vi "data-logging-test.vi"() -> ()   [LabVIEW 2023]
panel:
  out "error IO":errorcluster
  out "Datapoint 1":i32
  in  "Log File Name":path=path "log-00"
  in  "Start":bool
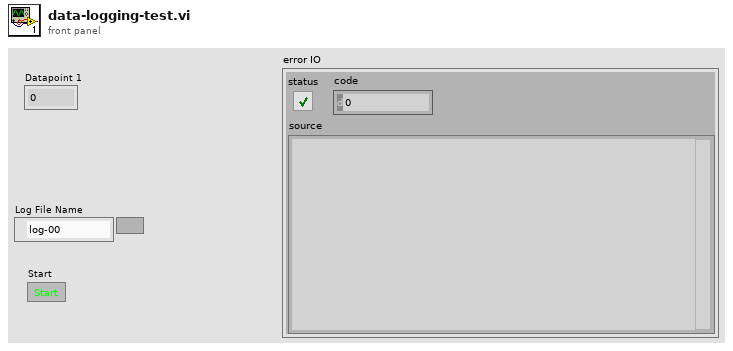
[diagram p1: front panel]
types:
  T1 = enum16{"open", "replace", "create", "open or create", "replace or create", "replace or create with confirmation"}
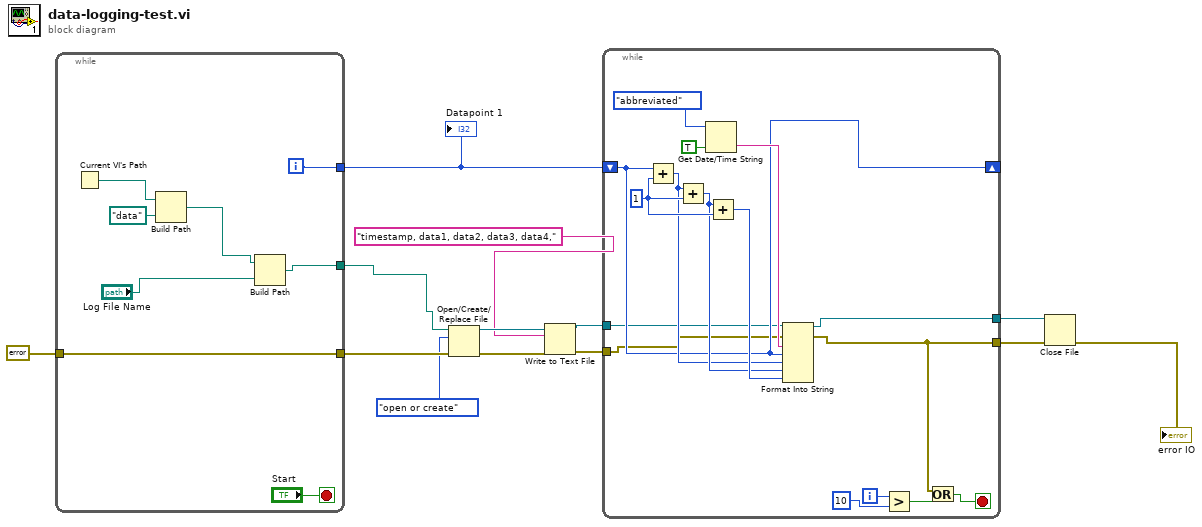
[diagram p0: block diagram]
diagram:
  n1 = while {
    tunnel: [w18] -> w10
    tunnel: errorcluster {"status"=FALSE, "code"=0, "source"=""} ("error in") -> [w18]
    tunnel: [w17] -> w6
    tunnel: [w13] -> w1
    i -> [w17]
    stop <- "Start" stop-if-true
    n2 = Current VI's Path() -> (path=w19:path)
    n3 = Build Path(base path=w19, name or relative path=path "data") -> (appended path=w15:path)
    n4 = Build Path(base path=w15, name or relative path="Log File Name") -> (appended path=w13:path)
  }
  "Datapoint 1" <- w6
  n5 = Open/Create/Replace File(file path (use dialog)=w1, error in=w10, operation (0:open)=T1."open or create") -> (refnum out=w9:refnum<file>, error out=w12:errorcluster)  [unwired: 3 in, 1 out]
  n6 = Write to Text File(file (use dialog)=w9, text="timestamp, data1, data2, data3, data4,", error in=w12) -> (refnum out=w8:refnum<file>, error out=w7:errorcluster)  [unwired: 1 in, 1 out]
  n7 = while {
    tunnel: w8 -> [w26]
    tunnel: w7 -> [w25]
    shift-right: [w27] -> _
    shift-left: w6 -> [w27]
    tunnel: [w21] -> w5
    tunnel: [w24] -> w4
    i -> [w36]
    stop <- w22 stop-if-true
    w34 = 1 ("y")
    n8 = Add(x=w27, y=w34) -> (x+y=w31:i32)
    n9 = Add(x=w31, y=w34) -> (x+y=w32:i32)
    n10 = Get Date/Time String(date format (0)=enum16{"short", "long", "abbreviated"}."abbreviated", want seconds? (F)=TRUE) -> (time string=w30:string)  [unwired: 1 in, 1 out]
    n11 = Add(x=w32, y=w34) -> (x+y=w33:i32)
    n12 = Format Into String(initial string=w26, error in=w25, w30, w27, w31, w32, w33) -> (resulting string=w24:refnum<file>, error out=w21:errorcluster)  [unwired: 1 in]
    n13 = Greater?(x=w36, y=10) -> (0:w23:bool)
    n14 = Or(x=w21, y=w23) -> (x .or. y?=w22:bool)
  }
  "error IO" <- w5
  n15 = Close File(refnum=w4, error in=w5) -> ()  [unwired: 2 out]
